vi "GetVariablesFromTarget.vi"(7 "PSP URL(ni.var.psp://)":string="ni.var.psp://", 8 "error in (no error)":errorcluster, 11 "IP Address String in":string) -> (0 "error out":errorcluster, 2 "AllVariables[]":refnum<k21>[](array[refnum]), 3 "IP Address String out":string)   [LabVIEW 2017, in "Shared Variables CD 2.0 Configuration.lvlib"]
uses:
  Shared Variables CD 2.0 Configuration.lvlib
  <resource>/objmgr/ni.var.rc
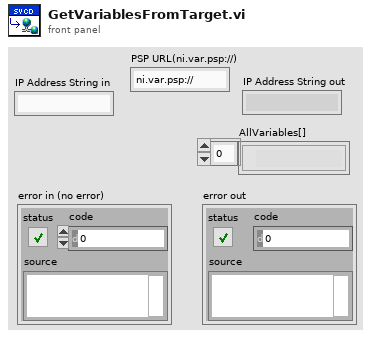
[diagram p1: front panel]
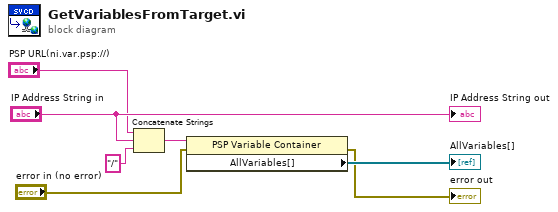
[diagram p0: block diagram]
diagram:
  n1 = Concatenate Strings("PSP URL(ni.var.psp://)", "IP Address String in", "/" ("string")) -> (w1:string)
  n2 = property class="PSP Variable Container"(reference=w1, error in="error in (no error)") -> (error out=→"error out":errorcluster, "AllVariables[]"=→"AllVariables[]":refnum<k21>[])  [unwired: 1 out]
  "IP Address String out" <- "IP Address String in"
